vi "_func_zip_vna_wmg.vi"(1 "destination path in zip":path caption="Zip文件目标路径", 2 "source file path":path caption="源文件路径", 3 "target":path caption="目标") -> (0 "error out":errorcluster caption="错误输出")   [LabVIEW 2011]
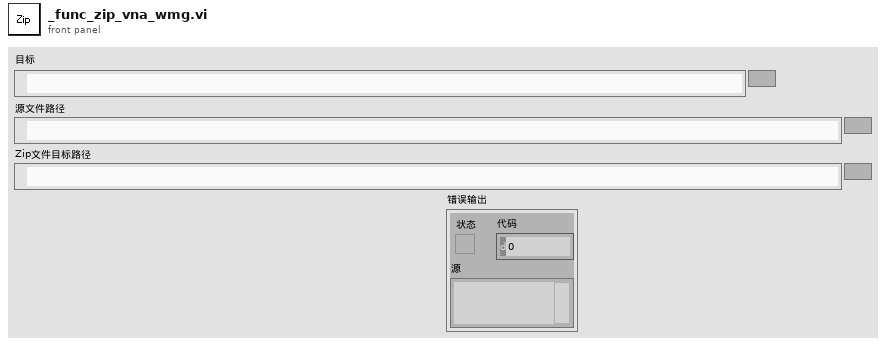
[diagram p1: front panel]
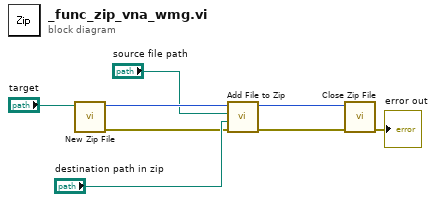
[diagram p0: block diagram]
diagram:
  n1 = call <vilib>:"New Zip File.vi"("target"="target") -> ("error out"=w3:errorcluster, "zip file out"=w8:i64)  [unwired: 4 in, 1 out]
  n2 = call <vilib>:"Add File to Zip.vi"("error in (no error)"=w3, "destination path in zip"="destination path in zip", "source file path"="source file path", "zip file in"=w8) -> ("error out"=w2:errorcluster, "zip file out"=w4:i64)  [unwired: 6 in]
  n3 = call <vilib>:"Close Zip File.vi"("error in (no error)"=w2, "zip file in"=w4) -> ("error out"=→"error out":errorcluster)  [unwired: 5 in]
